vi "get write location projection.vi"(10 "current volume":T1={"min x"=-1638, "deltaX"=41.0, "num x"=79, "max x"=1601, "min y"=-1638, "deltaY"=41.0, "num y"=80, "max y"=1642, "num z"=30, "num voxels"=189600, "voxels read"=0, "volume num"=0}, 11 "line":T2) -> (1 "zy insert point":u32, 2 "zx insert point":u32, 3 "xy insert point":u32)   [LabVIEW 2010]
uses:
  line_info.ctl
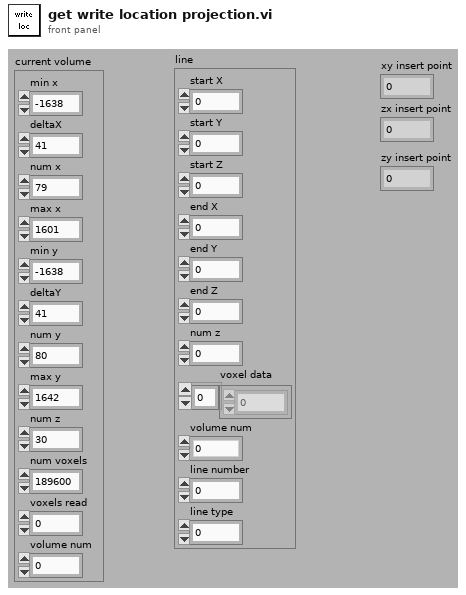
[diagram p1: front panel]
types:
  T1 = cluster{"min x":i16, "deltaX":dbl, "num x":u32, "max x":i16, "min y":i16, "deltaY":dbl, "num y":u32, "max y":i16, "num z":u32, "num voxels":u32, "voxels read":u32, "volume num":u32}
  T2 = typedef "line_info.ctl" = cluster{"start X":i16, "start Y":i16, "start Z":i16, "end X":i16, "end Y":i16, "end Z":i16, "num z":u8, "voxel data":u32[], "volume num":u32, "line number":u16, "line type":u16}
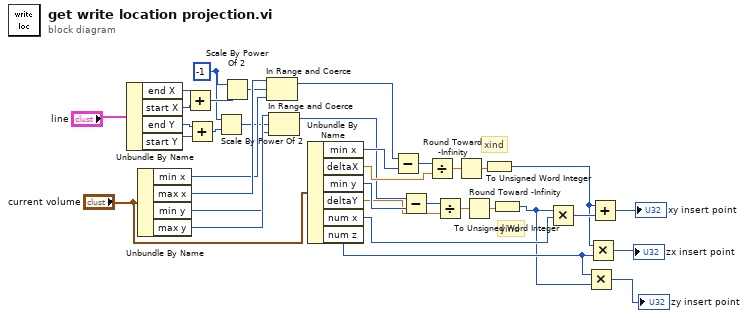
[diagram p0: block diagram]
diagram:
  w1 = -1 ("n")
  # "yind"
  # "xind"
  n1 = Unbundle By Name("line") -> ("end X"=w27:i16, "start X"=w26:i16, "end Y"=w25:i16, "start Y"=w24:i16)
  n2 = Unbundle By Name("current volume") -> ("min x"=w28:i16, "max x"=w29:i16, "min y"=w30:i16, "max y"=w31:i16)
  n3 = Add(x=w27, y=w26) -> (x+y=w23:i16)
  n4 = Add(x=w25, y=w24) -> (x+y=w22:i16)
  n5 = Scale By Power Of 2(n=w1, x=w22) -> (x*2^n=w20:i16)
  n6 = Scale By Power Of 2(n=w1, x=w23) -> (x*2^n=w21:i16)
  n7 = In Range and Coerce(upper limit=w29, x=w21, lower limit=w28) -> (coerced(x)=w32:i16)  [unwired: 1 out]
  n8 = In Range and Coerce(upper limit=w31, x=w20, lower limit=w30) -> (coerced(x)=w11:i16)  [unwired: 1 out]
  n9 = Unbundle By Name("current volume") -> ("min x"=w33:i16, "deltaX"=w17:dbl, "min y"=w12:i16, "deltaY"=w10:dbl, "num x"=w9:u32, "num z"=w4:u32)
  n10 = Subtract(x=w32, y=w33) -> (x-y=w19:i16)
  n11 = Subtract(x=w11, y=w12) -> (x-y=w15:i16)
  n12 = Divide(x=w19, y=w17) -> (x/y=w18:dbl)
  n13 = Divide(x=w15, y=w10) -> (x/y=w14:dbl)
  n14 = Round Toward -Infinity(1:w18) -> (0:w16:dbl)
  n15 = Round Toward -Infinity(1:w14) -> (0:w13:dbl)
  n16 = To Unsigned Word Integer(number=w16) -> (unsigned 16bit integer=w6:u16)
  n17 = To Unsigned Word Integer(number=w13) -> (unsigned 16bit integer=w3:u16)
  n18 = Multiply(x=w3, y=w9) -> (x*y=w8:u32)
  n19 = Multiply(x=w4, y=w3) -> (x*y=→"zy insert point":u32)
  n20 = Multiply(x=w6, y=w4) -> (x*y=→"zx insert point":u32)
  n21 = Add(x=w6, y=w8) -> (x+y=→"xy insert point":u32)
